vi "dsdll_output_write_int16.vi"(5 "volume (1: don't change volume)":i32=1 min=-10000 max=1 step=1, 6 "looped mode (true)":bool=TRUE, 7 "play (true)":bool=TRUE, 8 "error in":errorcluster, 9 "transpose (false)":bool, 10 "int16 samples":i16[][](array[numeric]), 11 "dsdll instance in":T1={"dsdll path"=path "E:/LVprog/DirectSoundDLL/dsdll.dll", "dsdll handle"=[], "output devices"=[], "capture devices"=[]}) -> (0 "error out":errorcluster, 3 "dsdll instance out":T1)   [LabVIEW 2020, in "dsdll.lvlib"]
doc: "Call this to write sample data into the output device buffer. \nOptionally starts playback and sets volume. If the 'volume' input left unconnectged it does not change the volume. The range of the volume is {-10000 to 0} where -10000 is equal to -100dB and 0 is 0dB (full volume).\nThe 'looped mode' option enables playback of the waveform in an infinite loop. If set to false the waveform will be played just once.\n\nData are expected in signed 16-bit integer format (2D array).\nIf the 'transpose' input is false: rows = channels, columns = samples.\nIf 'transpose' is true: columns = channels; rows = samples."
uses:
  dsdll.lvlib
  dsdll_instance.ctl
  dsdll_device_record.ctl
panel:
  out "output array":i16[](array[numeric])
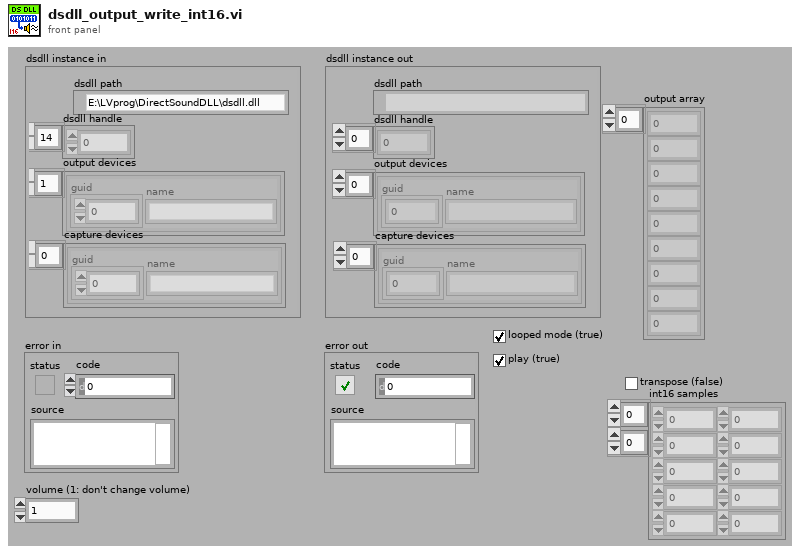
[diagram p1: front panel]
types:
  T1 = typedef "dsdll.lvlib/dsdll_instance.ctl" = cluster{"dsdll path":path, "dsdll handle":u8[], "output devices":T2[], "capture devices":T2[]}
  T2 = typedef "dsdll.lvlib/dsdll_device_record.ctl" = cluster{"guid":u8[], "name":string}
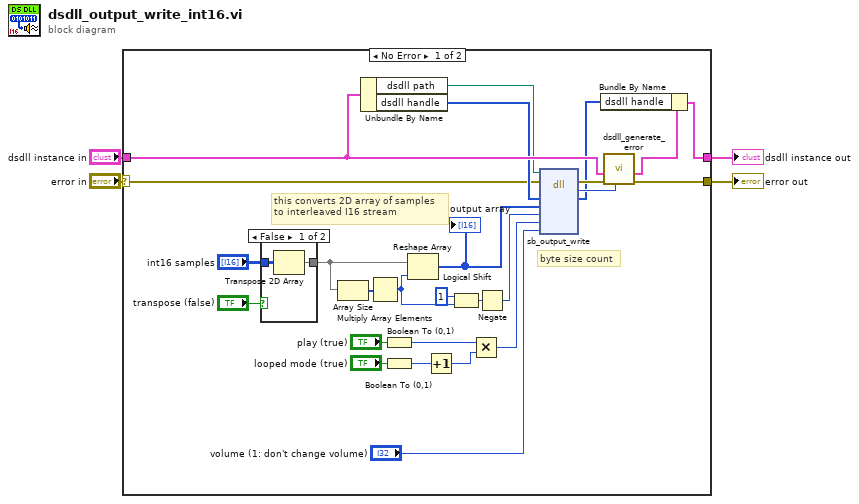
[diagram p0: block diagram]
diagram:
  n1 = case shown="No Error" "error in" {
    selector: "error in" -> [w21 w34]
    tunnel: "dsdll instance in" -> [w28 w35]
    tunnel: [w25 w34] -> w2
    tunnel: [w22 w35] -> w1
    frame No Error {
      # "this converts 2D array of samples\nto interleaved I16 stream"
      # "byte size count"
      n2 = case shown="False" "transpose (false)" {
        tunnel: [w32 w33] -> w14
        tunnel: "int16 samples" -> [w31 w33]
        frame False {
          n3 = Transpose 2D Array(2D array=w31) -> (transposed array=w32:i16[][])
        }
        frame True {
        }
      }
      n4 = Array Size(array=w14) -> (size(s)=w13:i32[])
      n5 = Unbundle By Name(w28) -> ("dsdll path"=w27:path, "dsdll handle"=w26:u8[])
      n6 = Multiply Array Elements(1:w13) -> (0:w11:i32)
      n7 = Boolean To (0,1)(Boolean="play (true)") -> (0, 1=w8:i16)
      n8 = Boolean To (0,1)(Boolean="looped mode (true)") -> (0, 1=w5:i16)
      n9 = Reshape Array(w14, w11) -> (w12:i16[])
      "output array" <- w12
      n10 = Increment(x=w5) -> (x+1=w9:i16)
      n11 = Logical Shift(y=i16 1, x=w11) -> (x << y=w17:i32)
      n12 = Multiply(x=w8, y=w9) -> (x*y=w7:i16)
      n13 = Negate(x=w17) -> (-x=w20:i32)
      n14 = dll-call lib="dsdll.dll" fn="sb_output_write" ("sb_get_handle_size()")(path in=w27, error in=w21, "handle"=w26, "data"=w12, "count"=w20, "play"=w7, "volume"="volume (1: don't change volume)") -> (error out=w30:errorcluster, "error"=w29:i32, "handle"=w23:u8[])  [unwired: 5 in, 1 out]
      n15 = call "dsdll_generate_error.vi"("error code"=w29, "error in"=w30, "dsdll instance in"=w28) -> ("error out"=w25:errorcluster, "dsdll instance out"=w24:T1)  [unwired: 6 in, 1 out]
      n16 = Bundle By Name(cluster=w24, "dsdll handle"=w23) -> (w22:T1)
    }
    frame Error {
    }
  }
  "error out" <- w2
  "dsdll instance out" <- w1
